vi "Ref Sample.vi"() -> ()   [LabVIEW 2024]
uses:
  <vilib>/Utility/file.llb/Read Delimited Spreadsheet (string).vi
  <vilib>/Utility/file.llb/Read Delimited Spreadsheet (DBL).vi
  <userlib>/_OpenG.lib/array/array.llb/Sort 2D Array (DBL)__ogtk.vi
  <userlib>/_OpenG.lib/array/array.llb/openg_array.lvlib
panel:
  out "XY Graph":T1(graph)
  out "Sorted Array out":dbl[][](array[numeric]) format="%.2f"
  out "first row":string[](array[string])
  out "all rows":dbl[][](array[numeric])
  in  "Data File":path
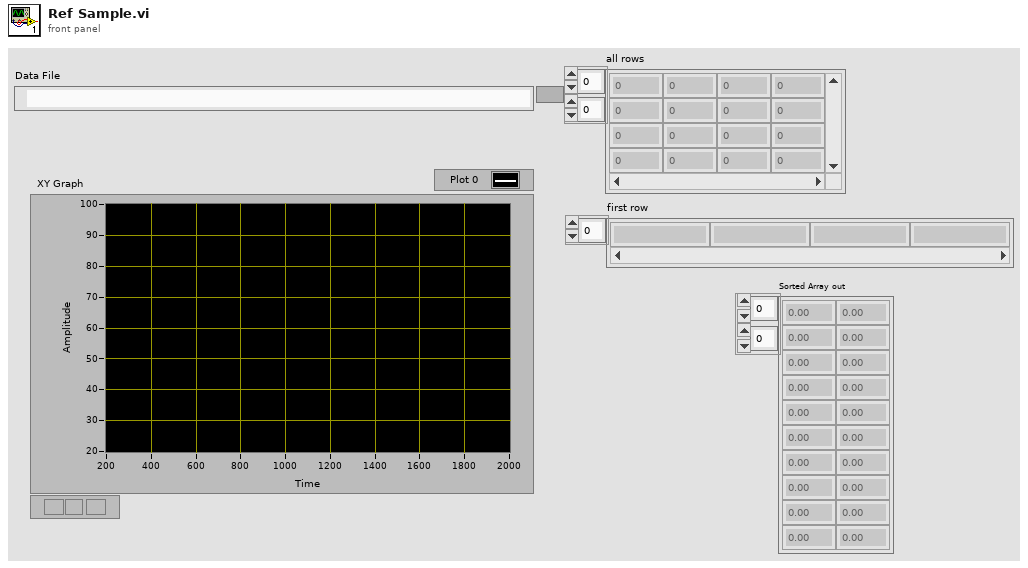
[diagram p1: front panel]
types:
  T1 = cluster{"Sorted Array out":dbl[], "Sorted Array out":dbl[]}
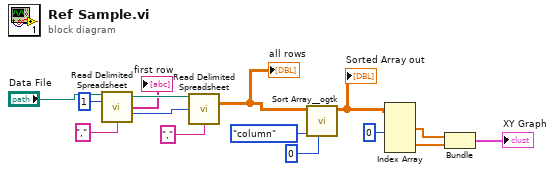
[diagram p0: block diagram]
diagram:
  n1 = call-poly <vilib>:"Read Delimited Spreadsheet.vi"("file path (dialog if empty)"="Data File", "number of rows (all:-1)"=1, "delimiter (\\t)"="," ("delimiter (\\t)")) -> ("new file path (Not A Path if cancelled)"=w14:path, "first row"=→"first row":string[], "mark after read (chars.)"=w11:i32)  [unwired: 7 in, 3 out]
  n2 = call-poly <vilib>:"Read Delimited Spreadsheet.vi"("file path (dialog if empty)"=w14, "start of read offset (chars.:0)"=w11, "delimiter (\\t)"="," ("delimiter (\\t)")) -> ("all rows"=w8:dbl[][])  [unwired: 7 in, 5 out]
  "all rows" <- w8
  n3 = call-poly <userlib>:"Sort Array__ogtk.vi"("Column/Row to Sort By"=u32 0, "Sort By in"=enum16{"row", "column"}."column", "Array in"=w8) -> ("Sorted Array out"=w5:dbl[][])  [unwired: 5 in, 3 out]
  "Sorted Array out" <- w5
  n4 = Index Array(array=w5, index (col) #1=0 ("disabled index (col)")) -> (element #1=w3:dbl[], element #2=w2:dbl[])  [unwired: 3 in]
  n5 = Bundle("Sorted Array out"=w3, "Sorted Array out"=w2) -> (→"XY Graph":T1)  [unwired: 1 in]
